vi "ReadDensity.vi"(0 "object in":refnum<class "CoriFlowBFS1Plus.lvclass">, 5 "error in (no error)":errorcluster) -> (14 "object out":refnum<class "CoriFlowBFS1Plus.lvclass">, 16 "Density_g_L":sgl, 19 "error out":errorcluster)   [LabVIEW 2021, in "CoriFlowBFS1Plus.lvclass"]
uses:
  CoriFlowBFS1Plus.lvclass
  CoriFlowBFS1Plus.lvclass/CoriFlowBFS1Plus.ctl
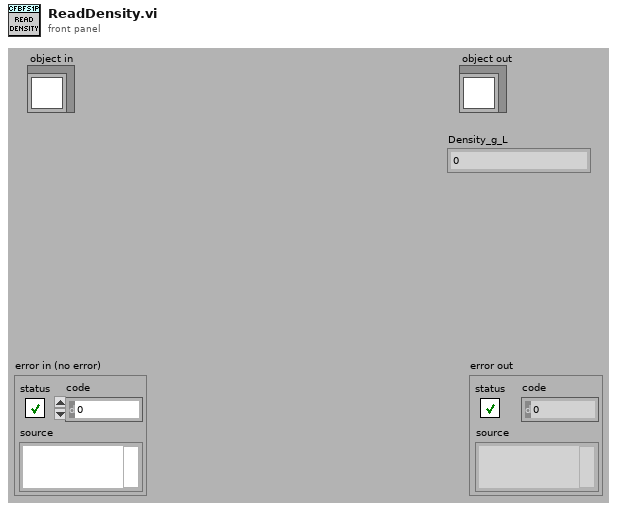
[diagram p1: front panel]
types:
  T1 = typedef "Z_BFS_type.ctl" = cluster{"VISA_Name":refnum<visa-resource-name>, "density_g_L":dbl, "Capacity":dbl, "Capacity units conversion":dbl}
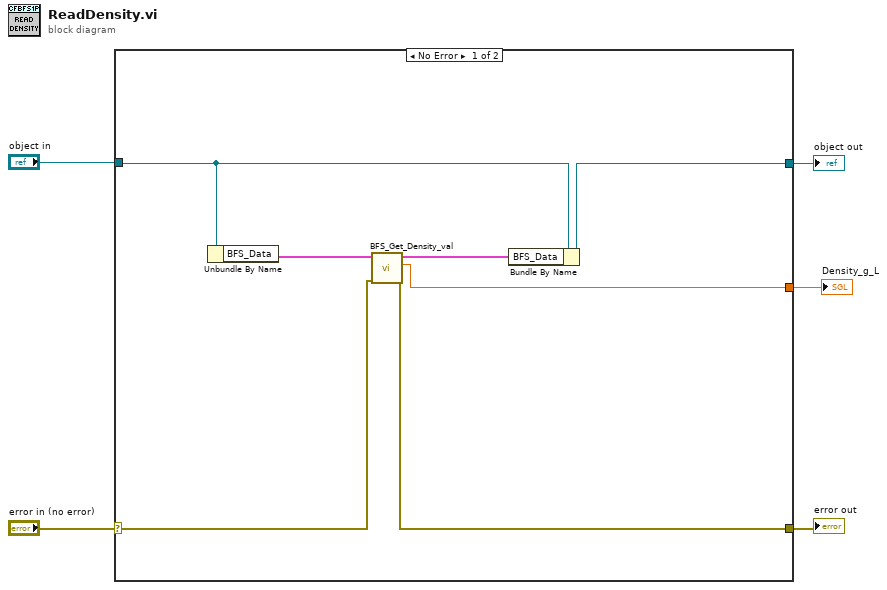
[diagram p0: block diagram]
diagram:
  n1 = case shown="No Error" "error in (no error)" {
    selector: "error in (no error)" -> [w7 w14]
    tunnel: [w6 w14] -> w4
    tunnel: [w11 w13] -> w2
    tunnel: "object in" -> [w12 w13]
    tunnel: [w8 _] -> w1
    frame No Error {
      n2 = Unbundle By Name(w12) -> ("BFS_Data"=w10:T1)
      n3 = call "BFS_Get_Density_val.vi"("error in (no error)"=w7, "BFS_type_In"=w10) -> ("error out"=w6:errorcluster, "Density_g_L"=w8:sgl, "BFS_type_Out"=w9:T1)  [unwired: 7 in]
      n4 = Bundle By Name(cluster=w12, "BFS_Data"=w9) -> (w11:refnum<class "CoriFlowBFS1Plus.lvclass">)
    }
    frame Error {
    }
  }
  "error out" <- w4
  "object out" <- w2
  "Density_g_L" <- w1
